vi "Hash.vi"(8 "error in (no error)":errorcluster, 10 "Message":string, 11 "MD5 in":refnum<class "MD5.lvclass">) -> (0 "error out":errorcluster, 2 "Hash":string, 3 "MD5 out":refnum<class "MD5.lvclass">)   [LabVIEW 2020, in "Crypto.lvlib" / "MD5.lvclass"]
uses:
  MD5.lvclass
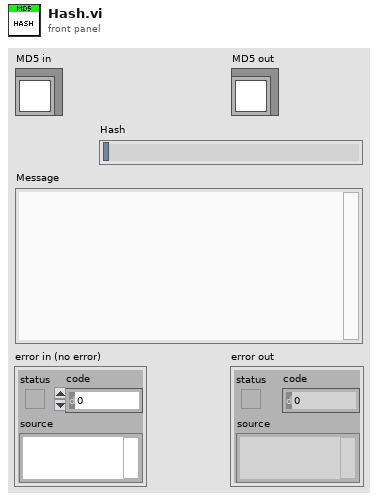
[diagram p1: front panel]
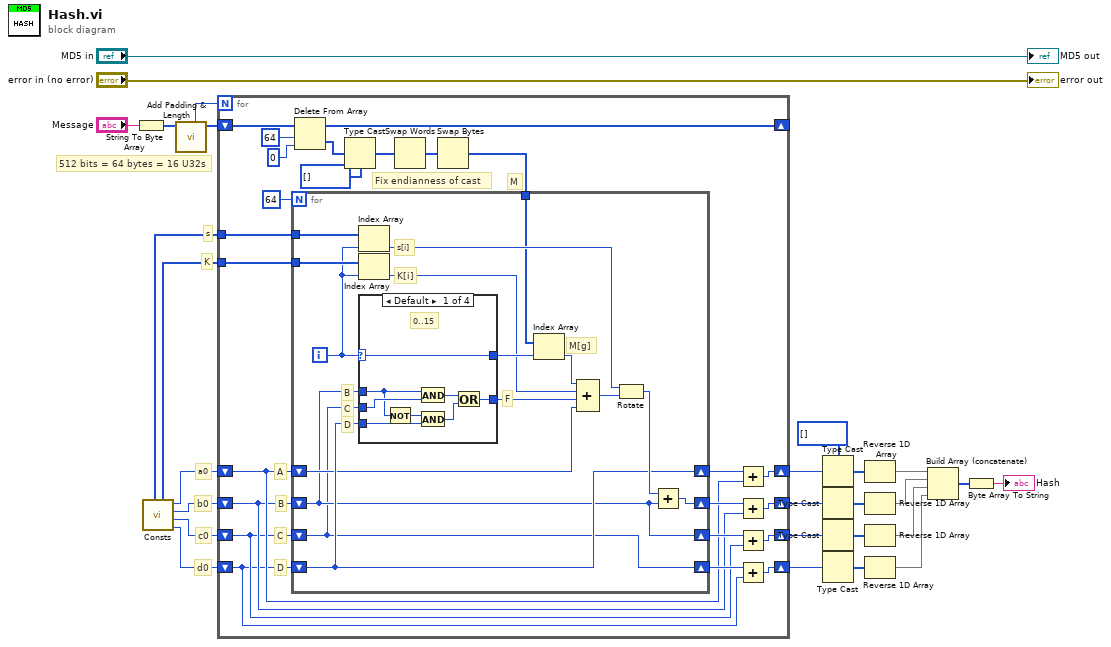
[diagram p0: block diagram]
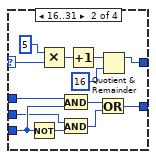
[diagram p2: hidden frame]
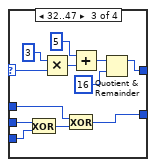
[diagram p3: hidden frame]
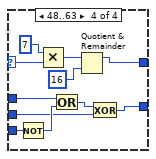
[diagram p4: hidden frame]
diagram:
  w13 = u8[] []
  # "512 bits = 64 bytes = 16 U32s"
  # "K"
  # "s"
  # "d0"
  # "c0"
  # "b0"
  # "a0"
  n1 = String To Byte Array(string="Message") -> (unsigned byte array=w24:u8[])
  n2 = call "Consts.vi"() -> ("d0"=w18:u32, "c0"=w19:u32, "b0"=w20:u32, "a0"=w21:u32, "K"=w16:u32[], "s"=w17:i16[])  [unwired: 6 in]
  n3 = call "Add Padding & Length.vi"("Data"=w24) -> ("Padded Data"=w22:u8[], "Blocks"=w23:i32)  [unwired: 9 in]
  n4 = for {
    N: w23 -> [_]
    shift-right: [w48] -> _
    shift-left: w22 -> [w51]
    shift-right: [w41] -> w15
    shift-left: w21 -> [w37]
    shift-right: [w40] -> w12
    shift-left: w20 -> [w36]
    shift-right: [w39] -> w11
    shift-left: w19 -> [w35]
    shift-right: [w38] -> w14
    shift-left: w18 -> [w34]
    tunnel: w17 -> [w33]
    tunnel: w16 -> [w32]
    # "Fix endianness of cast"
    # "D"
    # "C"
    # "B"
    # "A"
    # "M"
    n5 = Delete From Array(array=w51, length=64, index=0 ("length")) -> (deleted portion=w31:u8[], array with subset deleted=w48:u8[])
    n6 = Type Cast(type=u32[] [] ("length"), x=w31) -> (*(type *) &x=w30:u32[])
    n7 = Swap Words(1:w30) -> (0:w29:u32[])
    n8 = Swap Bytes(anything=w29) -> (byte swapped=w28:u32[])
    n9 = for {
      N: 64 -> [_]
      tunnel: w28 -> [w63]
      shift-right: [w62] -> w45
      shift-left: w37 -> [w54]
      shift-right: [w65] -> w44
      shift-left: w36 -> [w53]
      shift-right: [w53] -> w43
      shift-left: w35 -> [w52]
      shift-right: [w52] -> w42
      shift-left: w34 -> [w62]
      tunnel: w33 -> [w67]
      tunnel: w32 -> [w61]
      i -> [w56]
      # "K[i]"
      # "s[i]"
      # "F"
      # "D"
      # "C"
      # "B"
      # "M[g]"
      n10 = Index Array(array=w67, index=w56) -> (element=w66:i16)
      n11 = Index Array(array=w61, index=w56) -> (element=w55:u32)
      n12 = case shown="Default" w56 {
        selector: w56 -> [w75 w88 w91 w111]
        tunnel: w53 -> [w71 w82 w98 w105]
        tunnel: w52 -> [w72 w79 w100 w103]
        tunnel: w62 -> [w74 w81 w99 w106]
        tunnel: [w75 w83 w90 w108] -> w60
        tunnel: [w68 w76 w97 w101] -> w59
        frame Default {
          # "0..15"
          n13 = Not(x=w71) -> (.not. x?=w73:u32)
          n14 = And(x=w71, y=w72) -> (x .and. y?=w70:u32)
          n15 = And(x=w73, y=w74) -> (x .and. y?=w69:u32)
          n16 = Or(x=w70, y=w69) -> (x .or. y?=w68:u32)
        }
        frame 16..31 {
          n17 = Not(x=w81) -> (.not. x?=w80:u32)
          n18 = Multiply(x=5, y=w88) -> (x*y=w86:i32)
          n19 = And(x=w82, y=w81) -> (x .and. y?=w78:u32)
          n20 = And(x=w79, y=w80) -> (x .and. y?=w77:u32)
          n21 = Increment(x=w86) -> (x+1=w85:i32)
          n22 = Or(x=w78, y=w77) -> (x .or. y?=w76:u32)
          n23 = Quotient & Remainder(x=w85, y=16) -> (x-y*floor(x/y)=w83:i32)  [unwired: 1 out]
        }
        frame 32..47 {
          n24 = Exclusive Or(1:w99, 2:w100) -> (0:w96:u32)
          n25 = Multiply(x=3, y=w91) -> (x*y=w94:i32)
          n26 = Exclusive Or(1:w96, 2:w98) -> (0:w97:u32)
          n27 = Add(x=5, y=w94) -> (x+y=w93:i32)
          n28 = Quotient & Remainder(x=w93, y=16) -> (x-y*floor(x/y)=w90:i32)  [unwired: 1 out]
        }
        frame 48..63 {
          n29 = Not(x=w106) -> (.not. x?=w104:u32)
          n30 = Multiply(x=7, y=w111) -> (x*y=w109:i32)
          n31 = Or(x=w105, y=w104) -> (x .or. y?=w102:u32)
          n32 = Quotient & Remainder(x=w109, y=16) -> (x-y*floor(x/y)=w108:i32)  [unwired: 1 out]
          n33 = Exclusive Or(1:w103, 2:w102) -> (0:w101:u32)
        }
      }
      n34 = Index Array(array=w63, index=w60) -> (element=w58:u32)
      n35 = Compound Arithmetic op=ADD(w58, w55, w59, w54) -> (w57:u32)
      n36 = Rotate(1:w57, 2:w66) -> (0:w64:u32)
      n37 = Add(x=w64, y=w53) -> (x+y=w65:u32)
    }
    n38 = Add(x=w45, y=w37) -> (x+y=w41:u32)
    n39 = Add(x=w44, y=w36) -> (x+y=w40:u32)
    n40 = Add(x=w43, y=w35) -> (x+y=w39:u32)
    n41 = Add(x=w42, y=w34) -> (x+y=w38:u32)
  }
  n42 = Type Cast(type=w13, x=w15) -> (*(type *) &x=w10:u8[])
  n43 = Type Cast(type=w13, x=w12) -> (*(type *) &x=w9:u8[])
  n44 = Type Cast(type=w13, x=w11) -> (*(type *) &x=w8:u8[])
  n45 = Type Cast(type=w13, x=w14) -> (*(type *) &x=w7:u8[])
  n46 = Reverse 1D Array(array=w10) -> (reversed array=w2:u8[])
  n47 = Reverse 1D Array(array=w9) -> (reversed array=w5:u8[])
  n48 = Reverse 1D Array(array=w8) -> (reversed array=w4:u8[])
  n49 = Reverse 1D Array(array=w7) -> (reversed array=w3:u8[])
  n50 = Build Array (concatenate)(w2, w5, w4, w3) -> (w1:u8[])
  n51 = Byte Array To String(unsigned byte array=w1) -> (string=→"Hash":string)
  "error out" <- "error in (no error)"
  "MD5 out" <- "MD5 in"
